vi "Init Camera.vi"(8 "error in (no error)":errorcluster, 11 "CCDCamera in":refnum<class "CCDCamera.lvclass">) -> (0 "error out":errorcluster, 3 "CCDCamera out":refnum<class "CCDCamera.lvclass">)   [LabVIEW 2018, in "CCDCamera.lvclass"]
doc: "This VI initiates the camera, write to the class the CCD dimensions, the serial number , if the initialization is sucefull, and the temperature range."
uses:
  CCDCamera.lvclass
  CCDCamera.lvclass/CCDCamera.ctl
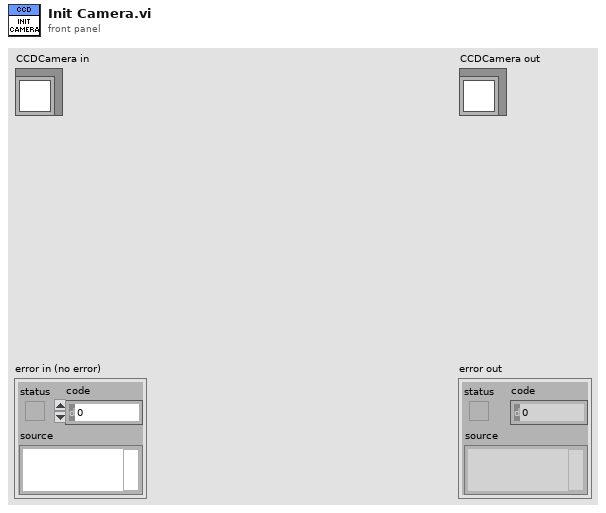
[diagram p1: front panel]
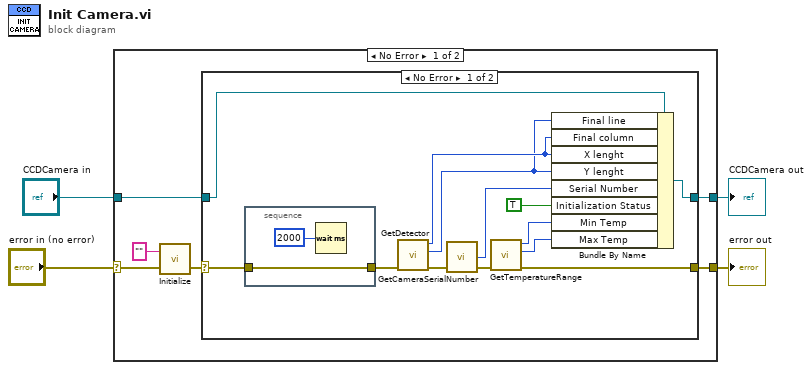
[diagram p0: block diagram]
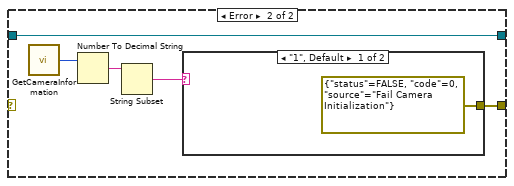
[diagram p2: hidden frame]
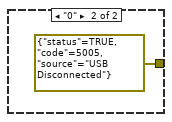
[diagram p3: hidden frame]
diagram:
  n1 = case shown="No Error" "error in (no error)" {
    selector: "error in (no error)" -> [w6 w34]
    tunnel: [w9 w34] -> w3
    tunnel: [w7 w33] -> w1
    tunnel: "CCDCamera in" -> [w5 w33]
    frame No Error {
      n2 = call <userlib>:"Initialize.vi"("error in (no error)"=w6, "directory (\"\")"="" ("directory (\"\")")) -> ("error out"=w10:errorcluster)  [unwired: 1 out]
      n3 = case shown="No Error" w10 {
        selector: w10 -> [w15 _]
        tunnel: [w16 w26] -> w9
        tunnel: w5 -> [w13 w30]
        tunnel: [w21 w30] -> w7
        frame No Error {
          n4 = stacked-sequence {
            tunnel: w15 -> [w24]
            tunnel: [w24] -> w14
            frame #0 {
              n5 = Wait (ms)(milliseconds to wait=u32 2000) -> ()  [unwired: 1 out]
            }
          }
          n6 = call <userlib>:"GetDetector.vi"("error in (no error)"=w14) -> ("error out"=w23:errorcluster, "ypixels"=w11:i32, "xpixels"=w12:i32)  [unwired: 3 in, 1 out]
          n7 = call <userlib>:"GetCameraSerialNumber.vi"("error in (no error)"=w23) -> ("error out"=w22:errorcluster, "number"=w17:i32)  [unwired: 2 in, 1 out]
          n8 = call <userlib>:"GetTemperatureRange.vi"("error in (no error)"=w22) -> ("error out"=w16:errorcluster, "maxTemp"=w19:i32, "minTemp"=w18:i32)  [unwired: 3 in, 1 out]
          n9 = Bundle By Name(cluster=w13, "Final line"=w11, "Final column"=w12, "X lenght"=w12, "Y lenght"=w11, "Serial Number"=w17, "Initialization Status"=TRUE, "Min Temp"=w18, "Max Temp"=w19) -> (w21:refnum<class "CCDCamera.lvclass">)
        }
        frame Error {
          n10 = call <userlib>:"GetCameraInformation.vi"() -> ("information"=w29:i32)  [unwired: 3 in, 2 out]
          n11 = Number To Decimal String(number=w29) -> (decimal integer string=w28:string)  [unwired: 1 in]
          n12 = String Subset(string=w28) -> (substring=w27:string)  [unwired: 2 in]
          n13 = case shown="\"1\", Default" w27 {
            tunnel: [errorcluster {"status"=FALSE, "code"=0, "source"="Fail Camera Initialization"} ("error out") errorcluster {"status"=TRUE, "code"=5005, "source"="USB Disconnected"} ("error out")] -> w26
            frame "1", Default {
            }
            frame "0" {
            }
          }
        }
      }
    }
    frame Error {
    }
  }
  "error out" <- w3
  "CCDCamera out" <- w1
